vi "initializeTPDO.vi"(8 "error in (no error)":errorcluster, 9 "PDO channel":u8(ring) items=["PDO 1", "PDO 2", "PDO 3", "PDO 4"], 10 "interface object in":refnum<k20>, 11 "MotorControllerClass in":refnum<class "MotorControllerClass.lvclass">) -> (0 "error out":errorcluster, 1 "TPDO object out":refnum<k20>, 2 "interface object out":refnum<k20>, 3 "MotorControllerClass out":refnum<class "MotorControllerClass.lvclass">)   [LabVIEW 2018, in "MotorControllerClass.lvclass"]
uses:
  BMS/MotorControllerClass.lvclass
  <vilib>/CANopenLib/CANOPEN.llb/CANopen TPDO Create.vi
  <vilib>/CANopenLib/CANOPEN.llb/CANopen TPDO Start.vi
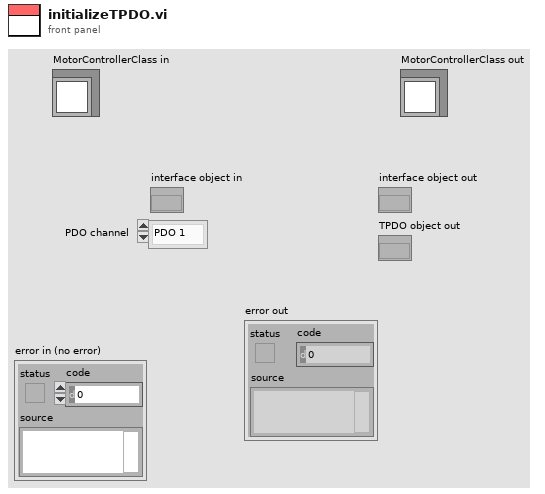
[diagram p1: front panel]
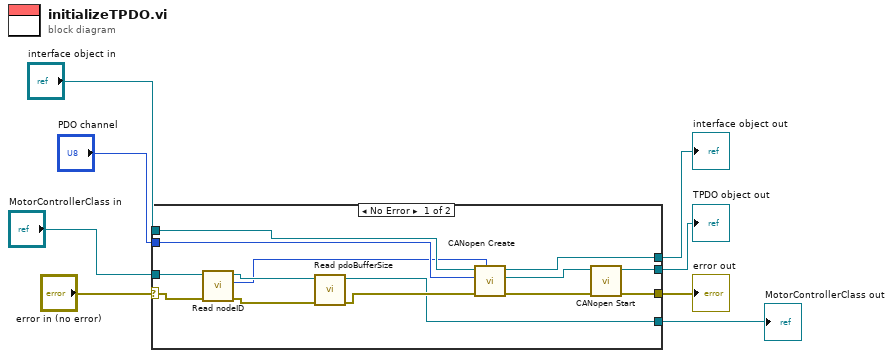
[diagram p0: block diagram]
diagram:
  n1 = case shown="No Error" "error in (no error)" {
    selector: "error in (no error)" -> [w12 w25]
    tunnel: [w16 w25] -> w7
    tunnel: "interface object in" -> [w22 w24]
    tunnel: "PDO channel" -> [w21 _]
    tunnel: [w20 w24] -> w4
    tunnel: [w18 _] -> w3
    tunnel: "MotorControllerClass in" -> [w15 w23]
    tunnel: [w9 w23] -> w1
    frame No Error {
      n2 = call-dynamic "Read nodeID.vi"("error in (no error)"=w12, "MotorControllerClass in"=w15) -> ("error out"=w11:errorcluster, "nodeID"=w13:u8, "MotorControllerClass out"=w14:refnum<class "MotorControllerClass.lvclass">)  [unwired: 7 in]
      n3 = call-dynamic "Read pdoBufferSize.vi"("error in (no error)"=w11, "MotorControllerClass in"=w14) -> ("error out"=w10:errorcluster, "MotorControllerClass out"=w9:refnum<class "MotorControllerClass.lvclass">)  [unwired: 7 in, 1 out]
      n4 = call-poly <vilib>:"CANopen Create.vi"("node-ID"=w13, "error in (no error)"=w10, "PDO channel"=w21, "interface object in"=w22) -> ("error out"=w17:errorcluster, "TPDO object out"=w19:refnum<k20>, "interface object out"=w20:refnum<k20>)  [unwired: 5 in]
      n5 = call-poly <vilib>:"CANopen Start.vi"("error in (no error)"=w17, "TPDO object in"=w19) -> ("error out"=w16:errorcluster, "TPDO object out"=w18:refnum<k20>)  [unwired: 8 in]
    }
    frame Error {
    }
  }
  "error out" <- w7
  "TPDO object out" <- w3
  "interface object out" <- w4
  "MotorControllerClass out" <- w1
